vi "FormatIDString.vi"(1 "ID String":string="00 00 00 01") -> (0 "ID":u32)   [LabVIEW 2011]
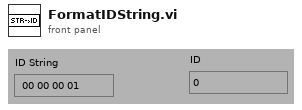
[diagram p1: front panel]
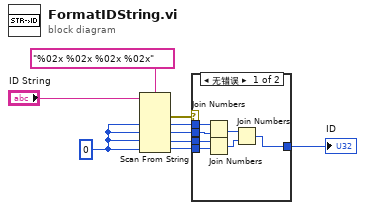
[diagram p0: block diagram]
diagram:
  w8 = u8 0
  n1 = Scan From String(format string="%02x %02x %02x %02x" ("格式字符串"), input string="ID String", default 1=w8, default 2=w8, default 3=w8, default 4=w8) -> (error out=w3:errorcluster, output 1=w2:u8, output 2=w1:u8, output 3=w6:u8, output 4=w5:u8)  [unwired: 2 in, 2 out]
  n2 = case shown="无错误" w3 {
    tunnel: w6 -> [w16 _]
    tunnel: w5 -> [w15 _]
    tunnel: [w10 _] -> w4
    tunnel: w2 -> [w14 _]
    tunnel: w1 -> [w13 _]
    frame No Error {
      n3 = Join Numbers(hi=w14, lo=w13) -> ((hi.lo)=w11:u16)
      n4 = Join Numbers(hi=w16, lo=w15) -> ((hi.lo)=w12:u16)
      n5 = Join Numbers(hi=w11, lo=w12) -> ((hi.lo)=w10:u32)
    }
    frame Error {
    }
  }
  "ID" <- w4
